vi "sub vi - Move Piezo Stage (Volts).vi"(10 "Volts":dbl min=0.0 format="%0.6f", 11 "Axis":u16(ring) items=["X", "Y", "Z"]) -> ()   [LabVIEW 2010]
uses:
  <vilib>/DAQmx/write.llb/DAQmx Write (Analog DBL 1Chan 1Samp).vi
  <vilib>/DAQmx/create/channels.llb/DAQmx Create Channel (AO-Voltage-Basic).vi
  <vilib>/daqmx/miscellaneous.llb/DAQmx Fill In Error Info.vi
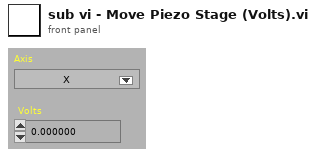
[diagram p1: front panel]
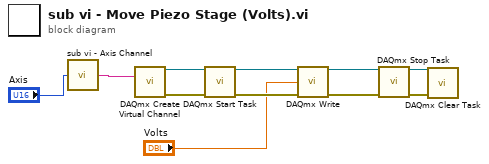
[diagram p0: block diagram]
diagram:
  n1 = call "sub vi - Axis Channel.vi"("Axis"="Axis") -> ("physical channels"=w3:tag)
  n2 = call-poly <vilib>:"DAQmx Create Virtual Channel.vi"("physical channels"=w3) -> ("task out"=w11:refnum<k21>, "error out"=w10:errorcluster)  [unwired: 8 in, 5 out]
  n3 = call <vilib>:"DAQmx Start Task.vi"("task/channels in"=w11, "error in"=w10) -> ("task out"=w7:refnum<k21>, "error out"=w4:errorcluster)  [unwired: 12 out]
  n4 = call-poly <vilib>:"DAQmx Write.vi"("task/channels in"=w7, "data"="Volts", "error in"=w4) -> ("task out"=w6:refnum<k21>, "error out"=w5:errorcluster)  [unwired: 1 in, 10 out]
  n5 = call <vilib>:"DAQmx Stop Task.vi"("task/channels in"=w6, "error in"=w5) -> ("task out"=w9:refnum<k21>, "error out"=w8:errorcluster)  [unwired: 12 out]
  n6 = call <vilib>:"DAQmx Clear Task.vi"("task in"=w9, "error in"=w8) -> ()  [unwired: 14 out]
